vi "test - Populate Variant with String (Double Quotes).vi"(8 "error in (no error)":errorcluster, 11 "TestCase in":refnum<class "Python Data Tools Tests.lvclass">) -> (0 "error out":errorcluster, 3 "TestCase out":refnum<class "Python Data Tools Tests.lvclass">)   [LabVIEW 2020, in "Python Data Tools Tests.lvclass"]
uses:
  Python Data Tools Tests.lvclass
  Python Data Tools Tests.lvclass/Python Data Tools Tests.ctl
  <vilib>/addons/_JKI Toolkits/VI Tester/TestCase.llb/TestCase.lvclass
  source/jki_python_data_tools.lvlib
  C:/Program Files/National Instruments/LabVIEW 2020/vi.lib/addons/_JKI Toolkits/VI Tester/TestCase.llb/TestCase.lvclass
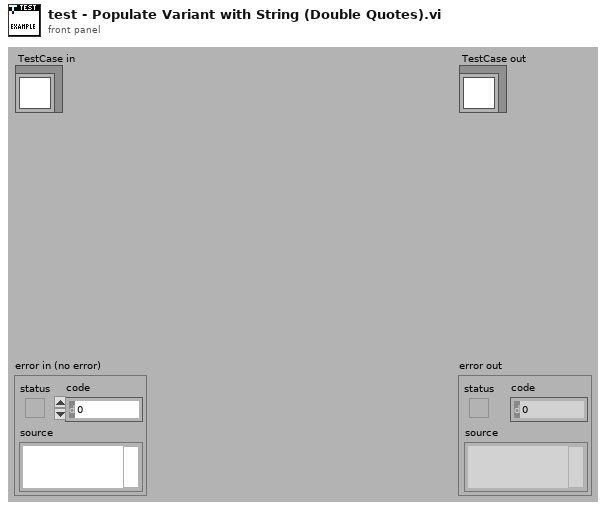
[diagram p1: front panel]
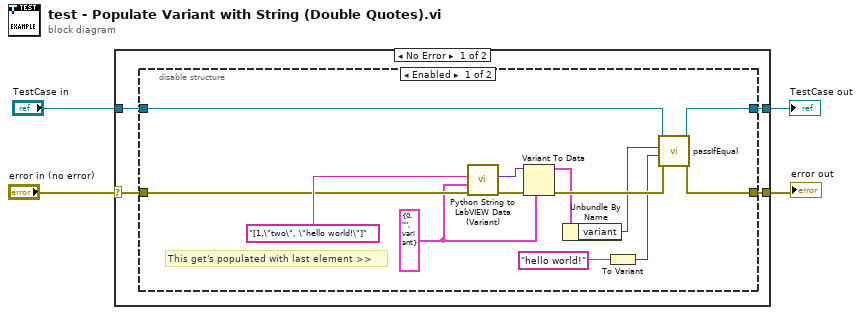
[diagram p0: block diagram]
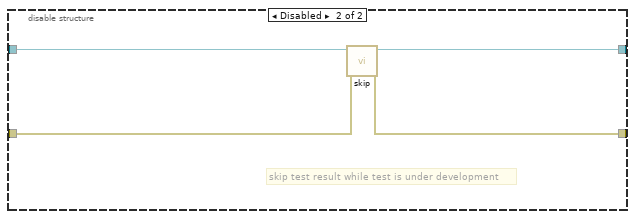
[diagram p2: hidden frame]
diagram:
  n1 = case shown="No Error" "error in (no error)" {
    selector: "error in (no error)" -> [w6 w27]
    tunnel: [w5 w27] -> w3
    tunnel: [w7 w26] -> w1
    tunnel: "TestCase in" -> [w8 w26]
    frame No Error {
      n2 = disable-structure shown="Enabled" {
        disable-tunnel: w8 -> [w21 w25]
        disable-tunnel: [w20 w22] -> w7
        disable-tunnel: w6 -> [w14 w24]
        disable-tunnel: [w19 w23] -> w5
        frame Enabled {
          w13 = cluster{i32, string, "variant":variant} {0, "", "variant"=variant}
          # "This get's populated with last element >>"
          n3 = call "Python String to LabVIEW Data (Variant).vi"("error in (no error)"=w14, "type"=w13, "Python String"="[1,\"two\", \"hello world!\"]") -> ("error out"=w16:errorcluster, "LabVIEW Data"=w17:variant)  [unwired: 7 in]
          n4 = Variant To Data(error in=w16, type=w13, Variant=w17) -> (data=w11:cluster{i32, string, "variant":variant}, error out=w15:errorcluster)
          n5 = Unbundle By Name(w11) -> ("variant"=w12:variant)
          n6 = To Variant(anything="hello world!") -> (Variant=w10:variant)
          n7 = call-dynamic "passIfEqual.vi"("error in (no error)"=w15, "y"=w10, "x"=w12, "TestCase in"=w21) -> ("error out"=w19:errorcluster, "TestCase out"=w20:refnum<class "Python Data Tools Tests.lvclass">)  [unwired: 6 in]
        }
        frame Disabled {
          # "skip test result while test is under development"
          n8 = call <vilib>:"skip.vi"("error in (no error)"=w24, "TestCase in"=w25) -> ("error out"=w23:errorcluster, "TestCase out"=w22:refnum<class "Python Data Tools Tests.lvclass">)  [unwired: 8 in]
        }
      }
    }
    frame Error {
    }
  }
  "error out" <- w3
  "TestCase out" <- w1
